vi "Channel Level.vi"(8 "error in (no error)":errorcluster, 11 "Node Ptr":T1 format="%.0x") -> (0 "error out":errorcluster)   [LabVIEW 2024, in "Embedded TDMS Logger System Explorer.lvlib"]
doc: "The Channel Page for user definition of the channel, allows the user to define:\n- Channel Name\n- Decimation\n- Meta Data to be tagged with the channel in the TDMS log\n\nNote: The Description is not logged in the TDMS file."
uses:
  Embedded TDMS Logger System Explorer.lvlib
  <vilib>/NI VeriStand/Custom Device API/Custom Device Item Ref.ctl
  <vilib>/NI VeriStand/Custom Device API/Get Item Property (Variant).vi
  <vilib>/NI VeriStand/Custom Device API/Get Item Property (I32).vi
  <vilib>/NI VeriStand/Custom Device API/Set Item Property (Variant).vi
  <vilib>/NI VeriStand/Custom Device API/Set Item Property (I32).vi
  <vilib>/NI VeriStand/Custom Device API/Custom Device API.lvlib
  Shared/File Classes/Meta Data.ctl
panel:
  in  "Decimation":i32
  in  "Channel Level Meta Data":string[][](table)
  in  "Specific Header":cluster{"Section Name":string}={"Section Name"="Specific Page Settings"}
  in  "General Header":cluster{"Section Name":string}={"Section Name"="General Page Settings"}
  in  "Description":string
  in  "Channel Name":string
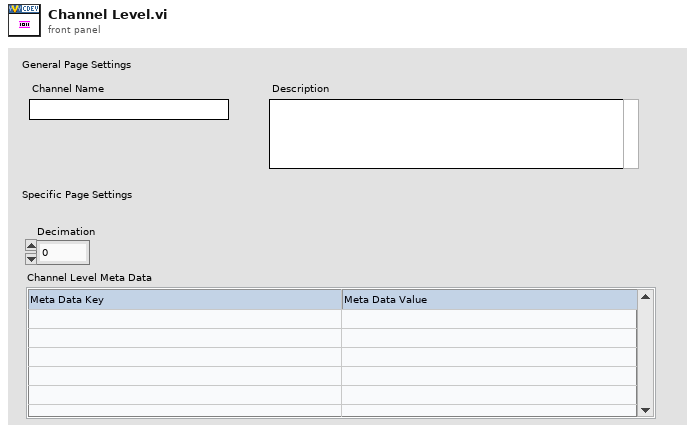
[diagram p1: front panel]
types:
  T1 = typedef "Custom Device API.lvlib/Custom Device Item Ref.ctl" = u64
  T2 = typedef "Meta Data.ctl" = cluster{"Key":string, "Value":string}
  T3 = typedef "Custom Device API.lvlib/Custom Device Item Info.ctl" = cluster{"Name":string, "Is Channel":bool, "GUID":string, "Is Waveform":bool}
  T4 = typedef "Custom Device API.lvlib/Custom Device Commands.ctl" = enum16{"Default", "Item renamed", "Shutdown", "Dynamic button pressed"}
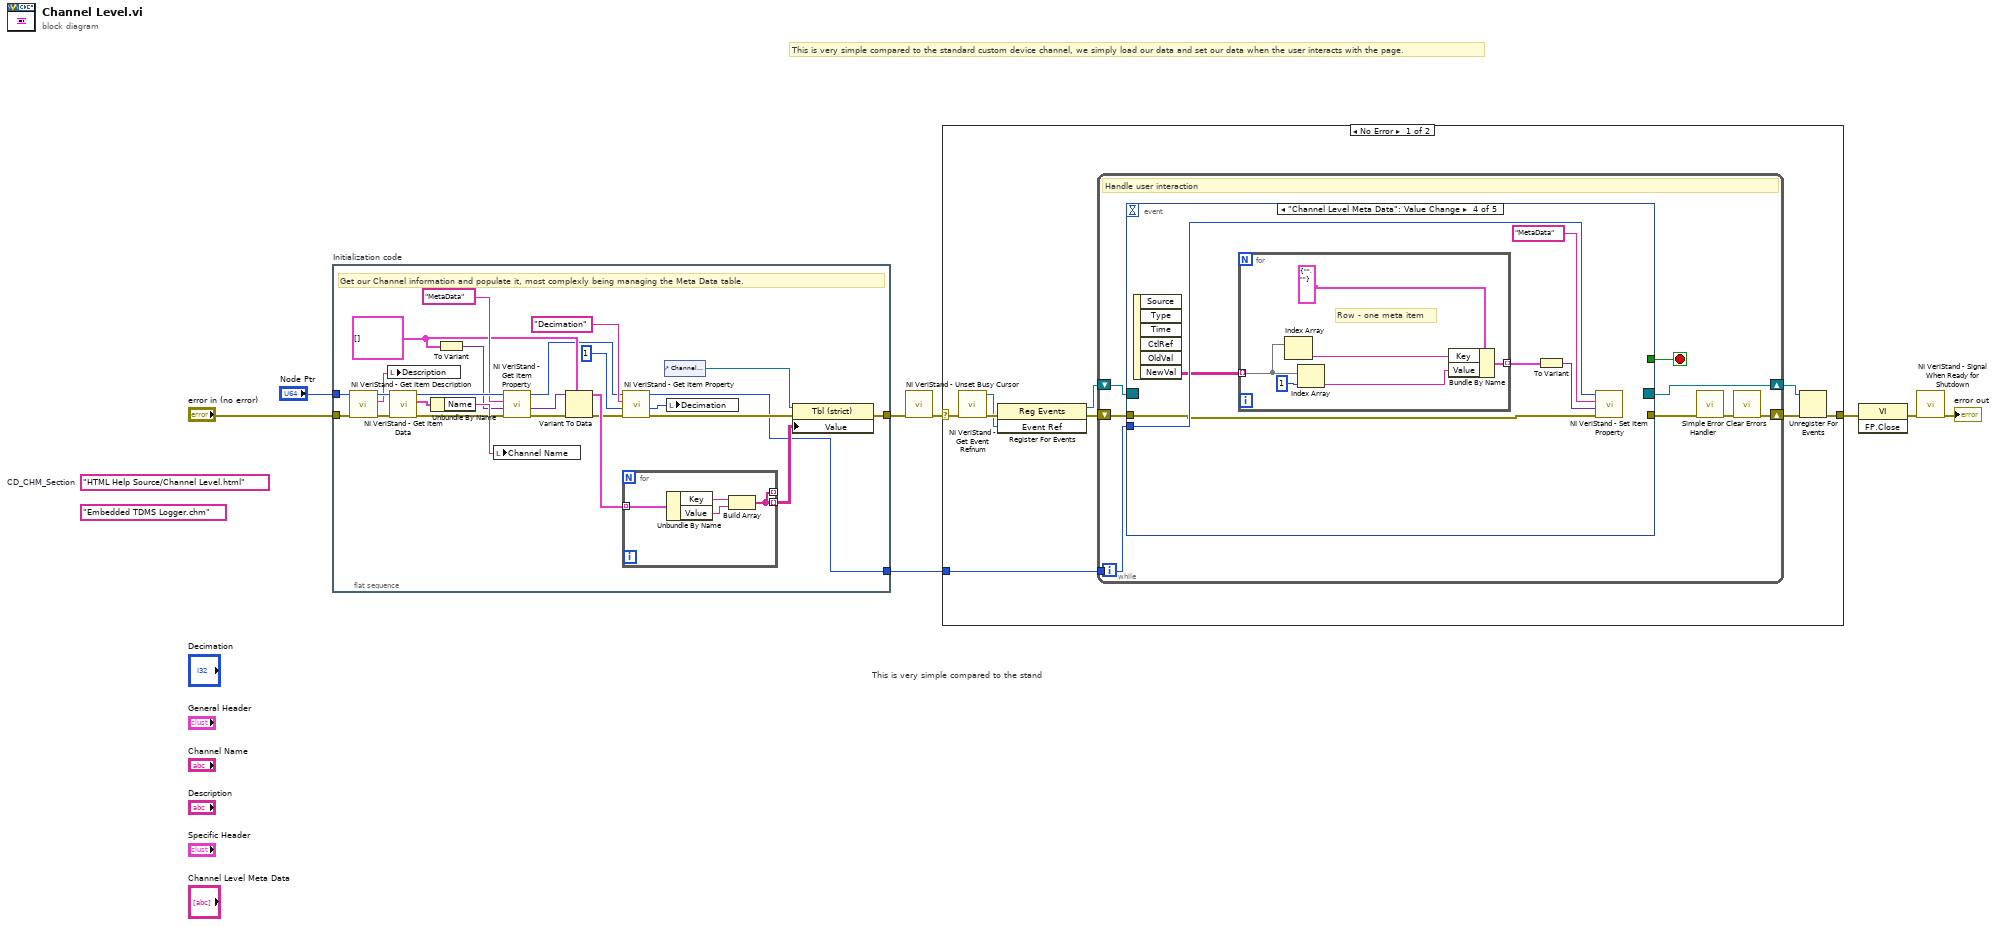
[diagram p0: block diagram]
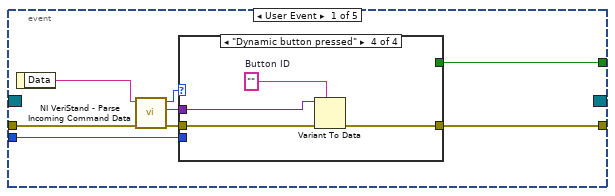
[diagram p2: hidden frame]
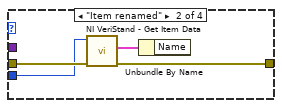
[diagram p4: hidden frame]
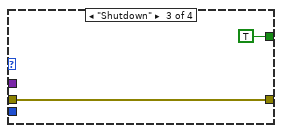
[diagram p5: hidden frame]
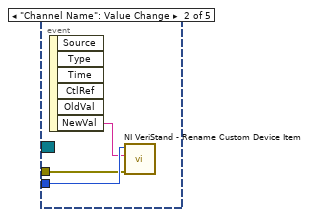
[diagram p6: hidden frame]
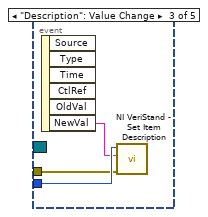
[diagram p7: hidden frame]
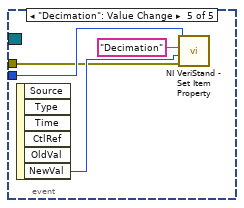
[diagram p8: hidden frame]
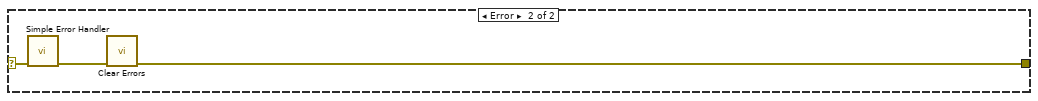
[diagram p9: hidden frame]
diagram:
  (unwired) "HTML Help Source/Channel Level.html"  # CD_CHM_Section
  (unwired) "Embedded TDMS Logger.chm" ("CD_CHM_FileName")
  # "This is very simple compared to the standard custom device channel, we simply load our data and set our data when the user interacts with the page."
  # "This is very simple compared to the stand"
  n1 = flat-sequence "Initialization code" {
    tunnel: "Node Ptr" -> [w16]
    tunnel: [w19] -> w3
    tunnel: [w9] -> w4
    tunnel: "error in (no error)" -> [w17]
    frame #0 {
      w22 = T2[] []
      # "Get our Channel information and populate it, most complexly being managing the Meta Data table."
      n2 = call <vilib>:"NI VeriStand - Get Item Description.vi"("error in (no error)"=w17, "Item Ref in"=w16) -> ("error out"=w32:errorcluster, "Description"=w29:string, "Item Ref out"=w33:T1)  [unwired: 7 out]
      n3 = local write "Description"(w29) -> ()
      n4 = call <vilib>:"NI VeriStand - Get Item Data.vi"("error in (no error)"=w32, "Item Ref in"=w33) -> ("error out"=w28:errorcluster, "Item Info"=w31:T3, "Item Ref out"=w27:T1)  [unwired: 7 out]
      n5 = Unbundle By Name(w31) -> ("Name"=w30:string)
      n6 = To Variant(anything=w22) -> (Variant=w25:variant)
      n7 = local write "Channel Name"(w30) -> ()
      n8 = call-poly <vilib>:"NI VeriStand - Get Item Property.vi"("error in (no error)"=w28, "Default Value"=w25, "Property Name"="MetaData", "Item Ref in"=w27) -> ("error out"=w24:errorcluster, "Value"=w23:variant, "Item Ref out"=w10:T1)  [unwired: 4 in, 1 out]
      n9 = Variant To Data(error in=w24, type=w22, Variant=w23) -> (data=w21:T2[], error out=w13:errorcluster)
      n10 = call-poly <vilib>:"NI VeriStand - Get Item Property.vi"("error in (no error)"=w13, "Default Value"=1, "Property Name"="Decimation", "Item Ref in"=w10) -> ("error out"=w11:errorcluster, "Value"=w15:i32, "Item Ref out"=w9:T1)  [unwired: 4 in, 1 out]
      n11 = for {
        tunnel: w21 -> [w37] mode=indexing
        tunnel: [w34] -> _ mode=indexing
        tunnel: [w34] -> w20 mode=indexing
        n12 = Unbundle By Name(w37) -> ("Key"=w36:string, "Value"=w35:string)
        n13 = Build Array(w36, w35) -> (w34:string[])
      }
      n14 = control-ref of="Channel Level Meta Data"() -> (w18:refnum<vi>)
      n15 = local write "Decimation"(w15) -> ()
      n16 = property class="Tbl (strict)"(reference=w18, error in=w11, "Value"=w20) -> (error out=w19:errorcluster)  [unwired: 1 out]
    }
  }
  n17 = call <vilib>:"NI VeriStand - Unset Busy Cursor.vi"("error in (no error)"=w3) -> ("error out"=w5:errorcluster)  [unwired: 10 out]
  n18 = case shown="No Error" w5 {
    selector: w5 -> [w38 w98]
    tunnel: [w43 w96] -> w8
    tunnel: w4 -> [w39 _]
    frame No Error {
      n19 = call <vilib>:"NI VeriStand - Get Event Refnum.vi"("error in (no error)"=w38) -> ("error out"=w46:errorcluster, "Event Ref"=w42:refnum<user-event>)  [unwired: 9 out]
      n20 = register-events(error in=w46, w42) -> (reference out=w40:refnum<event-registration>, error out=w41:errorcluster)  [unwired: 1 in]
      n21 = while {
        tunnel: w39 -> [w50]
        shift-right: [w47] -> w44
        shift-left: w41 -> [w53]
        shift-right: [w54] -> w45
        shift-left: w40 -> [w52]
        stop <- w51 stop-if-true
        # "Handle user interaction"
        n22 = event shown="[3] \"Channel Level Meta Data\": Value Change" {
          selector: w52 -> [_ _ _ _ _]
          dyn-events: [_ _ _ _ _] -> w54
          timeout: _ -> [_ _ _ _ _]
          tunnel: w53 -> [w62 w74 w78 w80 w92]
          tunnel: [w58 _ _ _ _] -> w51
          tunnel: [w57 _ _ _ _] -> w49
          tunnel: w50 -> [w56 w76 w79 w82 w94]
          event User Event {
            n23 = event-data() -> ("Data"=w61:string)  [unwired: 1 out]
            n24 = call <vilib>:"NI VeriStand - Parse Incoming Command Data.vi"("error in (no error)"=w62, "Incoming data"=w61) -> ("error out"=w60:errorcluster, "Outgoing data"=w55:variant, "Action"=w59:T4)  [unwired: 7 out]
            n25 = case shown="\"Dynamic button pressed\"" w59 {
              tunnel: w60 -> [w63 w67 w68 w73]
              tunnel: [_ _ TRUE _] -> w58
              tunnel: [w63 w64 w68 w70] -> w57
              tunnel: w56 -> [_ w66 _ _]
              tunnel: w55 -> [_ _ _ w72]
              frame "Default", Default {
              }
              frame "Item renamed" {
                n26 = call <vilib>:"NI VeriStand - Get Item Data.vi"("error in (no error)"=w67, "Item Ref in"=w66) -> ("error out"=w64:errorcluster, "Item Info"=w65:T3)  [unwired: 8 out]
                n27 = Unbundle By Name(w65) -> ()  [unwired: 1 out]
              }
              frame "Shutdown" {
              }
              frame "Dynamic button pressed" {
                w71 = ""  # Button ID
                n28 = Variant To Data(error in=w73, type=w71, Variant=w72) -> (error out=w70:errorcluster)  [unwired: 1 out]
              }
            }
          }
          event "Channel Name": Value Change {
            n29 = event-data() -> ("NewVal"=w75:string)  [unwired: 6 out]
            n30 = call <vilib>:"NI VeriStand - Rename Custom Device Item.vi"("error in (no error)"=w74, "New Name"=w75, "Item Ref in"=w76) -> ()  [unwired: 6 in, 3 out]
          }
          event "Description": Value Change {
            n31 = event-data() -> ("NewVal"=w77:string)  [unwired: 6 out]
            n32 = call <vilib>:"NI VeriStand - Set Item Description.vi"("error in (no error)"=w78, "Description"=w77, "Item Ref in"=w79) -> ()  [unwired: 6 in, 3 out]
          }
          event "Channel Level Meta Data": Value Change {
            n33 = event-data() -> ("NewVal"=w81:string[][])  [unwired: 6 out]
            n34 = for {
              tunnel: w81 -> [w90] mode=indexing
              tunnel: [w87] -> w85 mode=indexing
              # "Row - one meta item"
              n35 = Index Array(array=w90) -> (element=w88:string)  [unwired: 1 in]
              n36 = Index Array(array=w90, index=1) -> (element=w89:string)
              n37 = Bundle By Name(cluster=T2 {"Key"="", "Value"=""} ("Meta Data"), "Key"=w88, "Value"=w89) -> (w87:T2)
            }
            n38 = To Variant(anything=w85) -> (Variant=w84:variant)
            n39 = call-poly <vilib>:"NI VeriStand - Set Item Property.vi"("error in (no error)"=w80, "Value"=w84, "Property Name"="MetaData", "Item Ref in"=w82) -> ()  [unwired: 5 in, 3 out]
          }
          event "Decimation": Value Change {
            n40 = event-data() -> ("NewVal"=w93:i32)  [unwired: 6 out]
            n41 = call-poly <vilib>:"NI VeriStand - Set Item Property.vi"("error in (no error)"=w92, "Value"=w93, "Property Name"="Decimation", "Item Ref in"=w94) -> ()  [unwired: 5 in, 3 out]
          }
        }
        n42 = call <vilib>:"Simple Error Handler.vi"("error in (no error)"=w49) -> ("error out"=w48:errorcluster)  [unwired: 1 in, 7 out]
        n43 = call <vilib>:"Clear Errors.vi"("error in (no error)"=w48) -> ("error out"=w47:errorcluster)  [unwired: 1 in, 5 out]
      }
      n44 = Unregister For Events(event registration refnum=w45, error in=w44) -> (error out=w43:errorcluster)
    }
    frame Error {
      n45 = call <vilib>:"Simple Error Handler.vi"("error in (no error)"=w98) -> ("error out"=w97:errorcluster)  [unwired: 1 in, 7 out]
      n46 = call <vilib>:"Clear Errors.vi"("error in (no error)"=w97) -> ("error out"=w96:errorcluster)  [unwired: 1 in, 5 out]
    }
  }
  n47 = invoke class="VI" method="FP.Close"(error in=w8) -> (error out=w7:errorcluster)  [unwired: 2 in, 2 out]
  n48 = call <vilib>:"NI VeriStand - Signal When Ready for Shutdown.vi"("error in (no error)"=w7) -> ("error out"=→"error out":errorcluster)  [unwired: 10 out]
